vi "ZigZag to I32.vi"(11 "ZigZag I32":i32) -> (3 "sint32":i32)   [LabVIEW 2020, in "LV-Proto.lvlib"]
uses:
  LV-Proto.lvlib
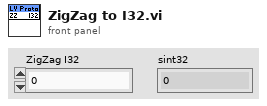
[diagram p1: front panel]
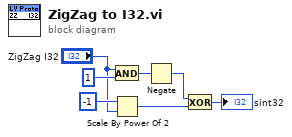
[diagram p0: block diagram]
diagram:
  n1 = And(x="ZigZag I32", y=1) -> (x .and. y?=w6:i32)
  n2 = Scale By Power Of 2(n=i16 -1, x="ZigZag I32") -> (x*2^n=w4:i32)
  n3 = Negate(x=w6) -> (-x=w3:i32)
  n4 = Exclusive Or(1:w4, 2:w3) -> (0:→"sint32":i32)
